vi "VMM_Main.vi"() -> ()   [LabVIEW 2020]
uses:
  <vilib>/vision/driver/IMAQdx.llb/IMAQdx Buffer Number Mode.ctl
  <vilib>/vision/driver/IMAQdx.llb/IMAQdx Acquisition Mode.ctl
  <extravilib>/ChannelInstances/High Speed Stream-a[.,.](u8).lvlib
  <vilib>/userDefined/High Color/IMAQdx.ctl
panel:
  out "HRME Image":T1(plugin-control)
  out "Zoomed Image":T1(plugin-control)
  in  "stop":bool
  in  "Session In":T2="cam2"
  out "Real-Time Mosaic":T1(plugin-control)
  # "Full-Resolution Mosaic"
  # "Zoomed in Mosaic"
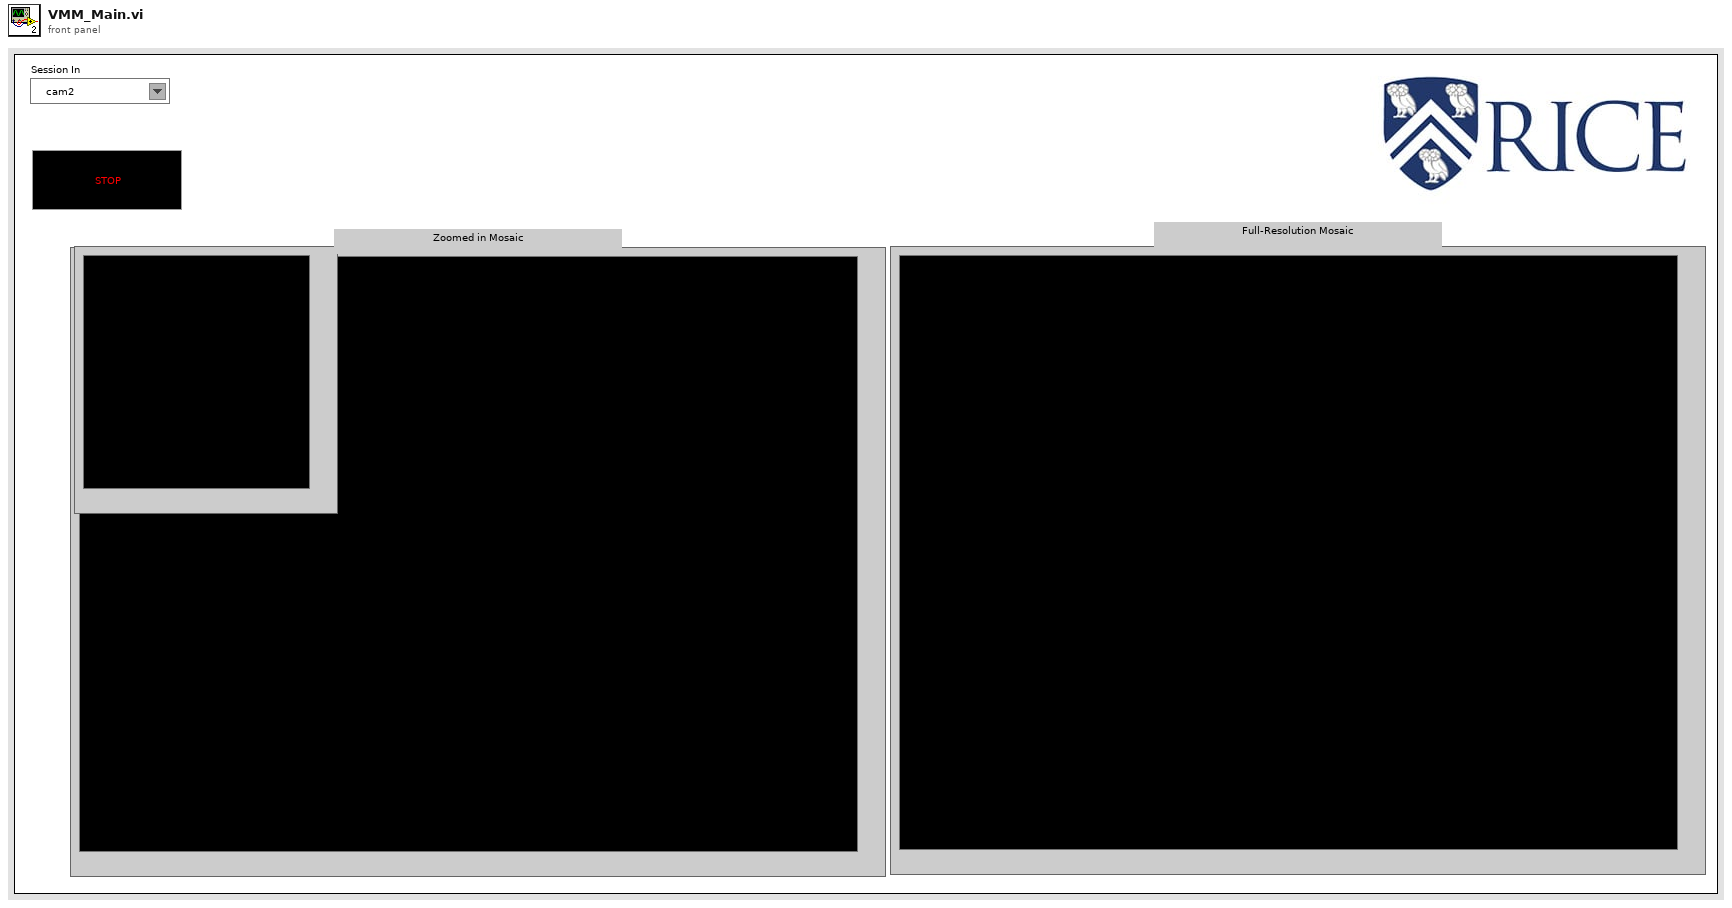
[diagram p1: front panel]
types:
  T1 = typedef "IMAQ Image.ctl" = refnum<image>
  T2 = typedef "IMAQdx.ctl" = refnum<k21>
  T3 = typedef "Image Type" = u32
  T4 = typedef "NI_Vision_Acquisition_Software.lvlib/IMAQdx Acquisition Mode.ctl" = enum32{"One Shot", "Continuous"}
  T5 = typedef "NI_Vision_Acquisition_Software.lvlib/IMAQdx Buffer Number Mode.ctl" = enum32{"Next", "Last", "Buffer Number", "Every", "Last New"}
  T6 = typedef "ROI Descriptor" = cluster{"Global Rectangle":i32[], "Contours":cluster{"ID":enum32{"External", "Internal"}, "Type":u32, "Coordinates":i32[]}[]}
  T7 = typedef "High Speed Stream-a[.,.](u8).lvlib/)Channel.ctl" = refnum<queue>
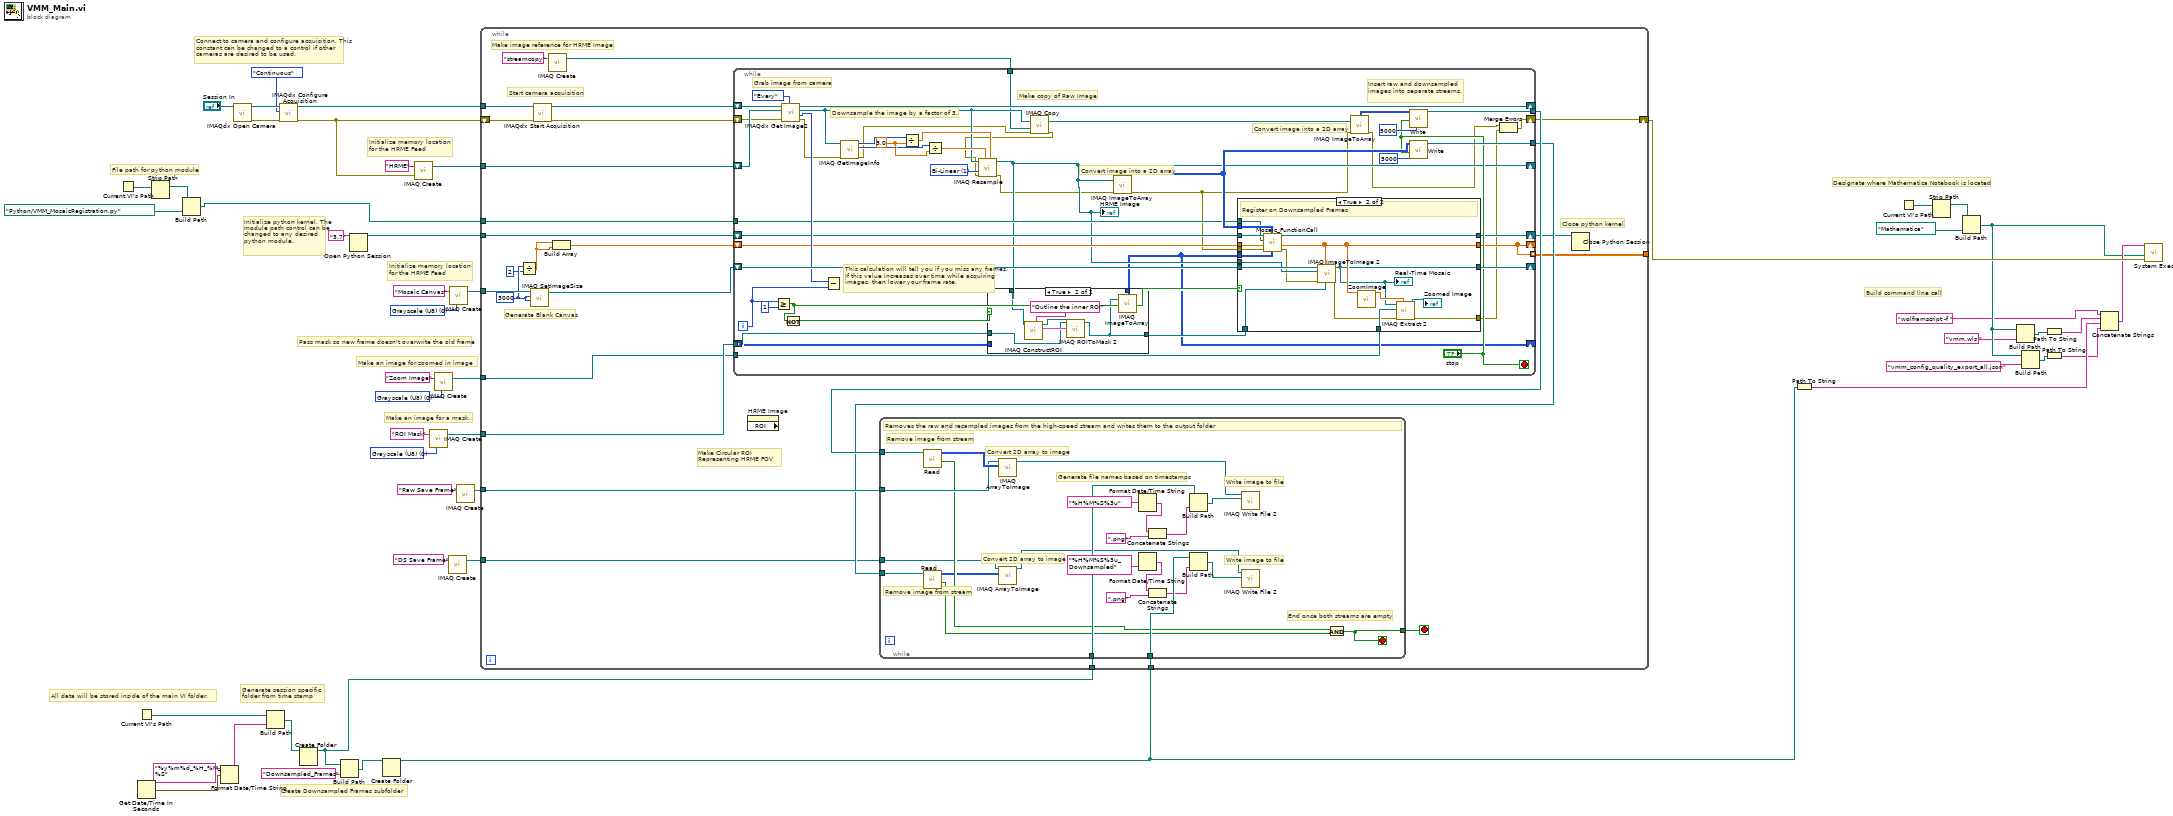
[diagram p0: block diagram]
diagram:
  w19 = T3 0 items=["Grayscale (U8)", "Grayscale (I16)", "Grayscale (SGL)", "Complex (CSG)", "RGB (U32)", "HSL (U32)", "RGB (U64)", "Grayscale (U16)"] ("Image Type")
  w25 = T3 0 items=["Grayscale (U8)", "Grayscale (I16)", "Grayscale (SGL)", "Complex (CSG)", "RGB (U32)", "HSL (U32)", "RGB (U64)", "Grayscale (U16)"] ("Image Type")
  w37 = T3 0 items=["Grayscale (U8)", "Grayscale (I16)", "Grayscale (SGL)", "Complex (CSG)", "RGB (U32)", "HSL (U32)", "RGB (U64)", "Grayscale (U16)"] ("Image Type")
  # "Build command line call"
  # "Designate where Mathematica Notebook is located"
  # "File path for python module"
  # "Make an image for zoomed in image"
  # "Generate session specific folder from time stamp"
  # "All data will be stored inside of the main VI folder."
  # "Pass mask so new frame doesn't overwrite the old frame"
  # "Make an image for a mask."
  # "Initialize memory location for the HRME Feed"
  # "Create Downsampled Frames subfolder"
  # "Initialize python kernel. The module path control can be changed to any desired python module."
  # "Initialize memory location for the HRME Feed"
  # "Connect to camera and configure acquisition. This constant can be changed to a control if other cameras are desired to be used."
  n1 = Current VI's Path() -> (path=w4:path)
  n2 = Get Date/Time In Seconds() -> (seconds since 1Jan1904=w35:timestamp)
  n3 = Current VI's Path() -> (path=w5:path)
  n4 = Strip Path(path=w4) -> (stripped path=w3:path)  [unwired: 1 out]
  n5 = Build Path(base path=w3, name or relative path=path "Python/VMM_MosaicRegistration.py" ("working directory")) -> (appended path=w1:path)
  n6 = Format Date/Time String(time format string (%c)="%y%m%d_%H_%M_%S", seconds (now)=w35) -> (date/time string=w34:string)  [unwired: 1 in]
  n7 = call <vilib>:"IMAQdx Open Camera.vi"("Session In"="Session In") -> ("error out"=w44:errorcluster, "Session Out"=w45:T2)  [unwired: 9 in]
  n8 = Build Path(base path=w5, name or relative path=w34) -> (appended path=w33:path)
  n9 = call <vilib>:"IMAQdx Configure Acquisition.vi"("error in"=w44, "Continuous?"=IMAQdx_Acquisition_Mode."Continuous", "Session In"=w45) -> ("error out"=w27:errorcluster, "Session Out"=w42:T2)  [unwired: 7 in]
  n10 = Create Folder(path (use dialog)=w33) -> (created path=w32:path)  [unwired: 2 in, 2 out]
  n11 = Build Path(base path=w32, name or relative path="Downsampled_Frames") -> (appended path=w31:path)
  n12 = Open Python Session(python version="3.7" ("Python version")) -> (session out=w47:refnum<k35>)  [unwired: 2 in, 1 out]
  n13 = Create Folder(path (use dialog)=w31) -> (created path=w24:path)  [unwired: 2 in, 2 out]
  n14 = call "IMAQ Create"("Image Name"="HRME", "error in (no error)"=w27) -> ("New Image"=w49:T1)  [unwired: 3 in, 1 out]
  n15 = call "IMAQ Create"("Image Name"="ROI Mask", "Image Type"=w25) -> ("New Image"=w17:T1)  [unwired: 3 in, 1 out]
  n16 = call "IMAQ Create"("Image Name"="Zoom Image", "Image Type"=w19) -> ("New Image"=w18:T1)  [unwired: 3 in, 1 out]
  n17 = call "IMAQ Create"("Image Name"="DS Save Frame") -> ("New Image"=w28:T1)  [unwired: 4 in, 1 out]
  n18 = call "IMAQ Create"("Image Name"="Mosaic Canvas", "Image Type"=w37) -> ("New Image"=w40:T1)  [unwired: 3 in, 1 out]
  n19 = call "IMAQ Create"("Image Name"="Raw Save Frame") -> ("New Image"=w38:T1)  [unwired: 4 in, 1 out]
  n20 = while {
    tunnel: w49 -> [w77]
    tunnel: w47 -> [w62]
    tunnel: w42 -> [w73]
    tunnel: w40 -> [w69]
    tunnel: w32 -> [w71]
    tunnel: w38 -> [w70]
    tunnel: w24 -> [w66]
    tunnel: w28 -> [w65]
    shift-right: [w54] -> w23
    shift-left: w27 -> [w75]
    tunnel: w1 -> [w61]
    tunnel: w17 -> [w53]
    tunnel: [w52] -> _
    tunnel: w18 -> [w51]
    stop <- w55 stop-if-true
    w59 = 3000 ("dimension size")
    # "Make Circular ROI Representing HRME FOV"
    # "Close python kernel"
    # "Generate Blank Canvas"
    # "Make image reference for HRME Image"
    # "Start camera acquisition"
    n21 = Divide(x=w59, y=2) -> (x/y=w57:dbl)
    n22 = call "IMAQ SetImageSize"("Y Resolution"=w59, "X Resolution"=w59, "Image"=w69) -> ("Image Out"=w68:T1)  [unwired: 2 in, 1 out]
    n23 = call <vilib>:"IMAQdx Start Acquisition.vi"("error in"=w75, "Session In"=w73) -> ("error out"=w74:errorcluster, "Session Out"=w72:T2)  [unwired: 8 in]
    n24 = call "IMAQ Create"("Image Name"="streamcopy") -> ("New Image"=w63:T1)  [unwired: 4 in, 1 out]
    n25 = Build Array(w57, w57) -> (w56:dbl[])
    n26 = while {
      shift-right: [w88] -> _
      shift-left: w77 -> [w120]
      tunnel: [w124] -> w76
      shift-right: [w109] -> _
      shift-left: w72 -> [w121]
      shift-right: [w95] -> _
      shift-left: w56 -> [w100]
      shift-right: [w117] -> _
      shift-left: w68 -> [w118]
      tunnel: [w106] -> w67
      shift-right: [w79] -> w54
      shift-left: w74 -> [w119]
      tunnel: w63 -> [w101]
      tunnel: w61 -> [w97]
      shift-right: [w96] -> w60
      shift-left: w62 -> [w98]
      tunnel: [w95] -> w52 mode=indexing
      tunnel: w53 -> [w89]
      tunnel: w51 -> [w93]
      shift-right: [w87] -> _
      shift-left: _ -> [w86]
      i -> [w116]
      stop <- "stop" stop-if-true
      w112 = 3.0 ("x/y")
      w113 = u32 1 items=["Zero Order", "Bi-Linear", "Quadratic", "Cubic Spline"] ("Interpolation Type")
      # "This calculation will tell you if you miss any frames. If this value increases over time while acquiring images, then lower your frame rate."
      # "Make copy of Raw Image"
      # "Convert image into a 2D array"
      # "Convert image into a 2D array"
      # "Insert raw and downsampled images into separate streams."
      # "Grab image from camera"
      # "Downsample the image by a factor of 3."
      n27 = Greater Or Equal?(x=w116, y=1) -> (x >= y?=w92:bool)
      n28 = call <vilib>:"IMAQdx Get Image2.vi"("Buffer Number Mode (Next)"=IMAQdx_Buffer_Number_Mode."Every", "error in"=w119, "Image In"=w120, "Session In"=w121) -> ("error out"=w85:errorcluster, "Buffer Number Out"=w108:u32, "Image Out"=w104:T1, "Session Out"=w109:T2)  [unwired: 4 in]
      n29 = Not(x=w92) -> (.not. x?=w91:bool)
      n30 = Subtract(x=w108, y=w116) -> ()  [unwired: 1 out]
      n31 = call "IMAQ GetImageInfo"("error in (no error)"=w85, "Image"=w104) -> ("error out"=w84:errorcluster, "Y Resolution"=w102:i32, "X Resolution"=w103:i32)  [unwired: 2 in, 5 out]
      n32 = Divide(x=w103, y=w112) -> (x/y=w111:dbl)
      n33 = Divide(x=w102, y=w112) -> (x/y=w110:dbl)
      n34 = call "IMAQ Copy"("error in (no error)"=w84, "Image Dst"=w101, "Image Src"=w104) -> ("error out"=w83:errorcluster, "Image Dst Out"=w94:T1)  [unwired: 3 in]
      n35 = call "IMAQ Resample"("X Resolution"=w111, "Y Resolution"=w110, "error in (no error)"=w83, "Interpolation Type"=w113, "Image Src"=w104) -> ("error out"=w82:errorcluster, "Image Dst Out"=w88:T1)  [unwired: 5 in]
      "HRME Image" <- w88
      n36 = case shown="True" w91 {
        tunnel: [w126 w128] -> w90
        tunnel: w89 -> [w126 w132]
        tunnel: w88 -> [_ w131]
        tunnel: [w125 w127] -> w87
        tunnel: w86 -> [w125 _]
        frame False {
        }
        frame True {
          n37 = call "IMAQ ConstructROI"("Prompt"="Outline the inner ROI", "Image"=w131) -> ("ROI Descriptor Out"=w133:T6, "Image Out (duplicate)"=w129:T1)  [unwired: 6 in, 2 out]
          n38 = call "IMAQ ROIToMask 2"("Image Model"=w129, "ROI Descriptor"=w133, "Image"=w132) -> ("Image Out"=w128:T1)  [unwired: 6 in, 2 out]
          n39 = call "IMAQ ImageToArray"("Image"=w128) -> ("Image Pixels (U8)"=w127:u8[][])  [unwired: 3 in, 4 out]
        }
      }
      n40 = call "IMAQ ImageToArray"("error in (no error)"=w82, "Image"=w88) -> ("error out"=w81:errorcluster, "Image Pixels (U8)"=w105:u8[][])  [unwired: 2 in, 3 out]
      n41 = case shown="True" w92 {
        tunnel: w105 -> [_ w154]
        tunnel: [w137 w145] -> w117
        tunnel: w118 -> [w137 w155]
        tunnel: [w136 w147] -> w95
        tunnel: w100 -> [w136 w153]
        tunnel: w98 -> [w135 w152]
        tunnel: w97 -> [_ w151]
        tunnel: [w135 w150] -> w96
        tunnel: w90 -> [_ w148]
        tunnel: w88 -> [_ w149]
        tunnel: w93 -> [_ w143]
        tunnel: w87 -> [_ w142]
        tunnel: [w134 w139] -> w78
        tunnel: w81 -> [w134 w138]
        frame False {
        }
        frame True {
          # "Register on Downsampled Frames"
          n42 = call "Mosaic_FunctionCall.vi"("Mask"=w142, "Current Frame"=w154, "error in (no error)"=w138, "Running Shift In"=w153, "module path"=w151, "session in"=w152) -> ("error out"=w141:errorcluster, "Running Shift Out"=w147:dbl[], "session out"=w150:refnum<k35>)  [unwired: 3 in]
          n43 = call "IMAQ ImageToImage 2"("Image Mask"=w148, "Offset Left/Top"=w147, "error in (no error)"=w141, "Image Src (Small)"=w149, "Image Src (Large)"=w155) -> ("error out"=w140:errorcluster, "Image Dst Out"=w145:T1)  [unwired: 5 in]
          "Real-Time Mosaic" <- w145
          n44 = call "ZoomImage.vi"("XY Shifts"=w147) -> ("Inner Crop Rect"=w146:dbl[])  [unwired: 10 in]
          n45 = call "IMAQ Extract 2"("Optional Rectangle"=w146, "error in (no error)"=w140, "Image Dst"=w143, "Image Src"=w145) -> ("error out"=w139:errorcluster, "Image Dst Out"=→"Zoomed Image":T1)  [unwired: 6 in]
        }
      }
      n46 = call "IMAQ ImageToArray"("error in (no error)"=w81, "Image"=w94) -> ("error out"=w80:errorcluster, "Image Pixels (U8)"=w114:u8[][])  [unwired: 2 in, 3 out]
      n47 = call <extravilib>:"Write.vi"("size (unlimited)"=5000, "last element? (F)"="stop", "element"=w114) -> ("channel"=w124:T7)  [unwired: 6 in, 2 out]
      n48 = call <extravilib>:"Write.vi"("size (unlimited)"=5000, "last element? (F)"="stop", "element"=w105) -> ("channel"=w106:T7)  [unwired: 6 in, 2 out]
      n49 = Merge Errors(w80, w78) -> (w79:errorcluster)
    }
    n50 = property on="HRME Image" props=["ROI"]() -> ()  [unwired: 2 in, 3 out]
    n51 = while {
      tunnel: w76 -> [w178]
      tunnel: [w170] -> w55
      tunnel: w71 -> [w176]
      tunnel: w70 -> [w175]
      tunnel: w67 -> [w173]
      tunnel: w66 -> [w174]
      tunnel: w65 -> [w169]
      stop <- w170 stop-if-true
      # "Remove image from stream"
      # "Remove image from stream"
      # "Convert 2D array to image"
      # "Convert 2D array to image"
      # "Write image to file"
      # "Write image to file"
      # "Generate file names based on timestamps"
      # "End once both streams are empty"
      # "Removes the raw and resampled images from the high-speed stream and writes them to the output folder"
      n52 = call <extravilib>:"Read.vi"("channel"=w178) -> ("done?"=w171:bool, "element"=w177:u8[][])  [unwired: 6 in, 3 out]
      n53 = call <extravilib>:"Read.vi"("channel"=w173) -> ("done?"=w172:bool, "element"=w168:u8[][])  [unwired: 6 in, 3 out]
      n54 = call "IMAQ ArrayToImage"("Image Pixels (U8)"=w177, "Image"=w175) -> ("Image Out"=w166:T1)  [unwired: 8 in, 1 out]
      n55 = call "IMAQ ArrayToImage"("Image Pixels (U8)"=w168, "Image"=w169) -> ("Image Out"=w157:T1)  [unwired: 8 in, 1 out]
      n56 = Format Date/Time String(time format string (%c)="%H%M%S%3u" ("Codec")) -> (date/time string=w163:string)  [unwired: 2 in]
      n57 = Format Date/Time String(time format string (%c)="%H%M%S%3u_Downsampled" ("Codec")) -> (date/time string=w160:string)  [unwired: 2 in]
      n58 = Concatenate Strings(w163, ".png" ("Codec")) -> (w162:string)
      n59 = Concatenate Strings(w160, ".png" ("Codec")) -> (w161:string)
      n60 = Build Path(base path=w176, name or relative path=w162) -> (appended path=w167:path)
      n61 = Build Path(base path=w174, name or relative path=w161) -> (appended path=w156:path)
      n62 = call-poly "IMAQ Write File 2"("File Path"=w167, "Image"=w166) -> ()  [unwired: 8 in, 2 out]
      n63 = call-poly "IMAQ Write File 2"("File Path"=w156, "Image"=w157) -> ()  [unwired: 8 in, 2 out]
      n64 = And(x=w171, y=w172) -> (x .and. y?=w170:bool)
    }
    n65 = Close Python Session(session in=w60) -> ()  [unwired: 1 in, 1 out]
  }
  n66 = Path To String(path=w24) -> (string=w22:string)
  n67 = Current VI's Path() -> (path=w16:path)
  n68 = Strip Path(path=w16) -> (stripped path=w15:path)  [unwired: 1 out]
  n69 = Build Path(base path=w15, name or relative path=path "Mathematica" ("working directory")) -> (appended path=w13:path)
  n70 = Build Path(base path=w13, name or relative path="vmm.wls " ("command line")) -> (appended path=w9:path)
  n71 = Build Path(base path=w13, name or relative path="vmm_config_quality_export_all.json" ("command line")) -> (appended path=w8:path)
  n72 = Path To String(path=w9) -> (string=w7:string)
  n73 = Path To String(path=w8) -> (string=w6:string)
  n74 = Concatenate Strings("wolframscript -f " ("command line"), w7, w22, w6) -> (w21:string)
  n75 = call <vilib>:"System Exec.vi"("error in (no error)"=w23, "working directory"=w13, "command line"=w21) -> ()  [unwired: 5 in, 4 out]
